vi "25StrToDecStr_dell.vi"(1 "input_str_hex":string) -> (0 "数值":i32)   [LabVIEW 2011]
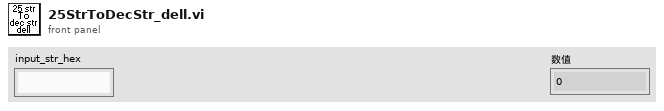
[diagram p1: front panel]
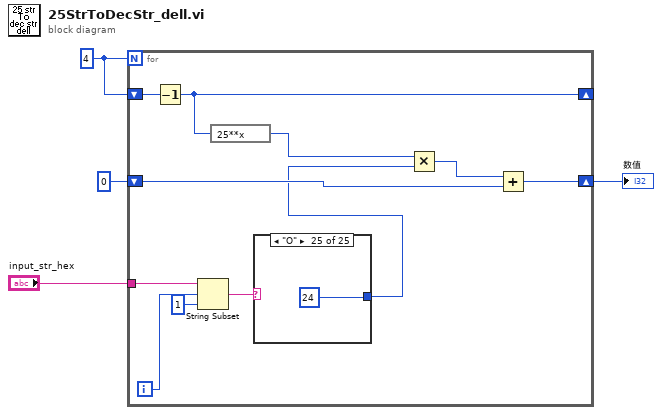
[diagram p0: block diagram]
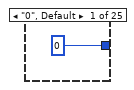
[diagram p2: hidden frame]
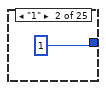
[diagram p3: hidden frame]
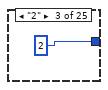
[diagram p4: hidden frame]
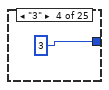
[diagram p5: hidden frame]
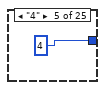
[diagram p6: hidden frame]
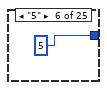
[diagram p7: hidden frame]
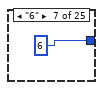
[diagram p8: hidden frame]
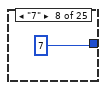
[diagram p9: hidden frame]
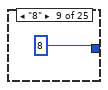
[diagram p10: hidden frame]
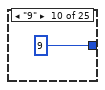
[diagram p11: hidden frame]
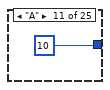
[diagram p12: hidden frame]
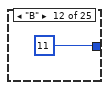
[diagram p13: hidden frame]
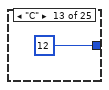
[diagram p14: hidden frame]
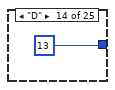
[diagram p15: hidden frame]
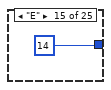
[diagram p16: hidden frame]
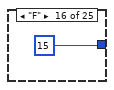
[diagram p17: hidden frame]
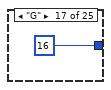
[diagram p18: hidden frame]
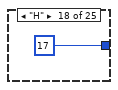
[diagram p19: hidden frame]
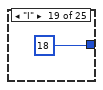
[diagram p20: hidden frame]
diagram:
  w4 = 4
  n1 = for {
    N: w4 -> [_]
    shift-right: [w6] -> _
    shift-left: w4 -> [w15]
    shift-right: [w12] -> w1
    shift-left: 0 -> [w13]
    tunnel: "input_str_hex" -> [w11]
    i -> [w10]
    n2 = Decrement(x=w15) -> (x-1=w6:i32)
    n3 = String Subset(string=w11, offset (0)=w10, length (rest)=1 ("长度（剩余）")) -> (substring=w8:string)
    n4 = expression code="25**x"(w6) -> (w5:i32)
    n5 = case shown="\"O\"" w8 {
      tunnel: [0 1 2 3 4 5 6 7 8 9 10 11 12 13 14 15 16 17 18 19 20 21 22 23 24] -> w7
      frame "0", Default {
      }
      frame "1" {
      }
      frame "2" {
      }
      frame "3" {
      }
      frame "4" {
      }
      frame "5" {
      }
      frame "6" {
      }
      frame "7" {
      }
      frame "8" {
      }
      frame "9" {
      }
      frame "A" {
      }
      frame "B" {
      }
      frame "C" {
      }
      frame "D" {
      }
      frame "E" {
      }
      frame "F" {
      }
      frame "G" {
      }
      frame "H" {
      }
      frame "I" {
      }
      frame "J" {
      }
      frame "K" {
      }
      frame "L" {
      }
      frame "M" {
      }
      frame "N" {
      }
      frame "O" {
      }
    }
    n6 = Multiply(x=w5, y=w7) -> (x*y=w14:i32)
    n7 = Add(x=w14, y=w13) -> (x+y=w12:i32)
  }
  "数值" <- w1
